vi "RisingEdgeDelay.vi"(7 "enable?":bool=TRUE, 10 "Deadtime (iterations)":u8=1, 11 "Input":bool) -> (3 "Output":bool)   [LabVIEW 2015, in "SPWM.lvlib"]
uses:
  SPWM.lvlib
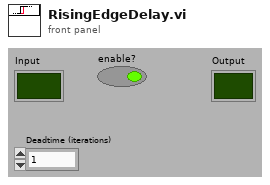
[diagram p1: front panel]
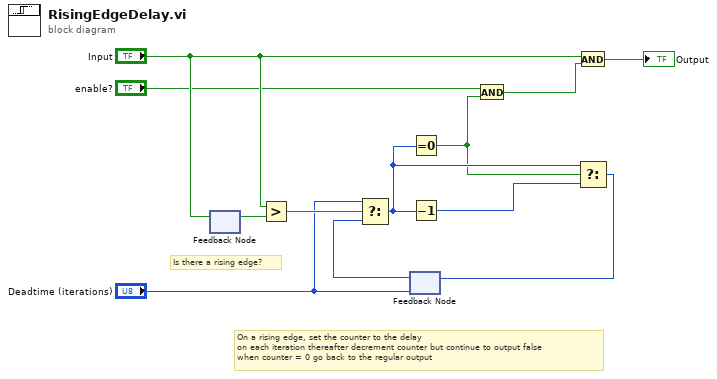
[diagram p0: block diagram]
diagram:
  # "Is there a rising edge?"
  # "On a rising edge, set the counter to the delay\non each iteration thereafter decrement counter but continue to output false\nwhen counter = 0 go back to the regular output"
  n1 = feedback-in #1("Input") -> ()
  n2 = feedback #1() -> (w8:bool)  [unwired: 1 in]
  n3 = Greater?(x="Input", y=w8) -> (0:w5:bool)
  n4 = feedback #2("Deadtime (iterations)") -> (w12:u8)
  n5 = Select(t="Deadtime (iterations)", s=w5, f=w12) -> (s? t:f=w7:u8)
  n6 = Equal To 0?(x=w7) -> (x = 0?=w6:bool)
  n7 = Decrement(x=w7) -> (x-1=w11:u8)
  n8 = And(x="enable?", y=w6) -> (x .and. y?=w4:bool)
  n9 = And(x="Input", y=w4) -> (x .and. y?=→"Output":bool)
  n10 = Select(t=w7, s=w6, f=w11) -> (s? t:f=w10:u8)
  n11 = feedback-in #2(w10) -> ()
